vi "solar_voy_def Export Type.vi"(0 "ID (F)":bool, 1 "CMD":enum8{"CMD", "TLM"}(ring), 5 "OFFSET (-1=APPEND)":i32=-1, 7 "TOTAL_SIZE (0)":i32, 9 "TYPE (BLOCK)":T1, 11 "EACH_SIZE (0=NoArray)":i32) -> (4 "COMMAND_DEF":string, 6 "TYPE_DEF":string)   [LabVIEW 2018]
doc: "This exports the parameter/item type to COSMOS item definition string. If OFFSET is -1, this uses the 'APPEND' definition tag. If EACH_SIZE > 0, this returns the 'ARRAY_' definition tag."
uses:
  solar_voy_def_ctl ITEM TYPE.ctl
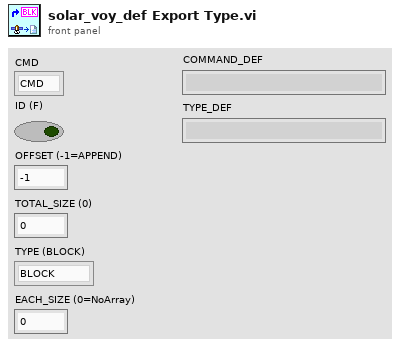
[diagram p1: front panel]
types:
  T1 = typedef "solar_voy_def_ctl ITEM TYPE.ctl" = enum8{"BLOCK", "INT", "UINT", "FLOAT", "STRING"}
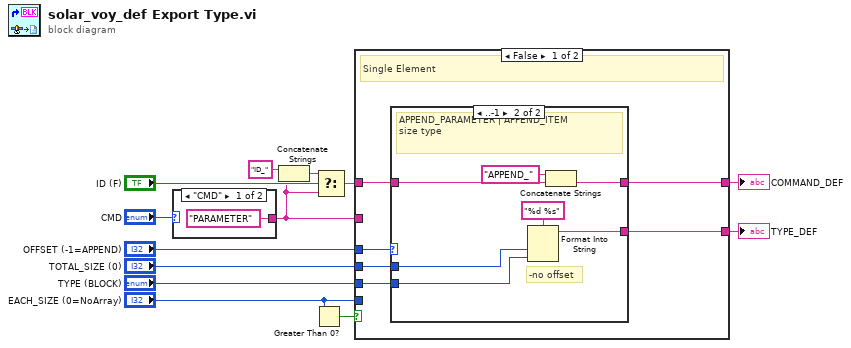
[diagram p0: block diagram]
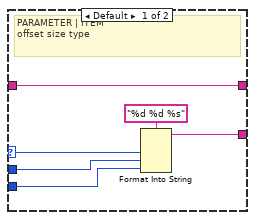
[diagram p2: hidden frame]
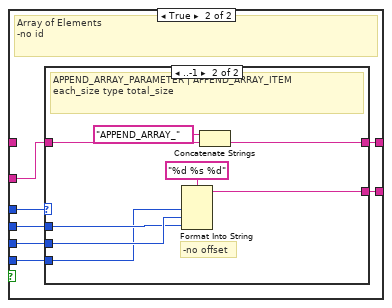
[diagram p3: hidden frame]
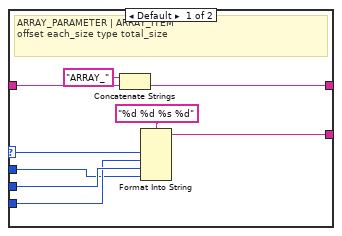
[diagram p4: hidden frame]
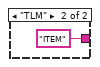
[diagram p5: hidden frame]
diagram:
  n1 = case shown="\"CMD\"" "CMD" {
    tunnel: ["PARAMETER" "ITEM"] -> w2
    frame "CMD" {
    }
    frame "TLM" {
    }
  }
  n2 = Concatenate Strings("ID_" ("string"), w2) -> (w9:string)
  n3 = Greater Than 0?(x="EACH_SIZE (0=NoArray)") -> (x > 0?=w4:bool)
  n4 = Select(t=w9, s="ID (F)", f=w2) -> (s? t:f=w8:string)
  n5 = case shown="False" w4 {
    tunnel: "TYPE (BLOCK)" -> [w21 w41]
    tunnel: [w20 w40] -> w13
    tunnel: w8 -> [w19 _]
    tunnel: [w18 w39] -> w7
    tunnel: "OFFSET (-1=APPEND)" -> [w17 w38]
    tunnel: "TOTAL_SIZE (0)" -> [w16 w37]
    tunnel: "EACH_SIZE (0=NoArray)" -> [_ w36]
    tunnel: w2 -> [_ w35]
    frame False {
      # "Single Element"
      n6 = case shown="..-1" w17 {
        selector: w17 -> [w25 _]
        tunnel: w21 -> [w23 w34]
        tunnel: [w22 w33] -> w20
        tunnel: w19 -> [w27 w30]
        tunnel: [w27 w29] -> w18
        tunnel: w16 -> [w24 w28]
        frame Default {
          # "PARAMETER | ITEM\noffset size type"
          n7 = Format Into String(format string="%d %d %s", w25, w24, w23) -> (resulting string=w22:string)  [unwired: 2 in, 1 out]
        }
        frame ..-1 {
          # "-no offset"
          # "APPEND_PARAMETER | APPEND_ITEM\nsize type"
          n8 = Format Into String(format string="%d %s", w28, w34) -> (resulting string=w33:string)  [unwired: 2 in, 1 out]
          n9 = Concatenate Strings("APPEND_" ("string"), w30) -> (w29:string)
        }
      }
    }
    frame True {
      # "Array of Elements\n-no id"
      n10 = case shown="..-1" w38 {
        selector: w38 -> [w49 _]
        tunnel: w41 -> [w48 w58]
        tunnel: [w47 w57] -> w40
        tunnel: w35 -> [w43 w54]
        tunnel: [w42 w53] -> w39
        tunnel: w37 -> [w45 w52]
        tunnel: w36 -> [w46 w51]
        frame Default {
          # "ARRAY_PARAMETER | ARRAY_ITEM\noffset each_size type total_size"
          n11 = Concatenate Strings("ARRAY_" ("string"), w43) -> (w42:string)
          n12 = Format Into String(format string="%d %d %s %d", w49, w46, w48, w45) -> (resulting string=w47:string)  [unwired: 2 in, 1 out]
        }
        frame ..-1 {
          # "-no offset"
          # "APPEND_ARRAY_PARAMETER | APPEND_ARRAY_ITEM\neach_size type total_size"
          n13 = Format Into String(format string="%d %s %d", w51, w58, w52) -> (resulting string=w57:string)  [unwired: 2 in, 1 out]
          n14 = Concatenate Strings("APPEND_ARRAY_" ("string"), w54) -> (w53:string)
        }
      }
    }
  }
  "TYPE_DEF" <- w13
  "COMMAND_DEF" <- w7
